vi "GT Set Capture Mode.vi"(8 "error in (no error)":errorcluster caption="错误输入（无错误）", 9 "mode":i16, 10 "encoder":i16, 11 "cardNum":i16) -> (0 "error out":errorcluster caption="错误输出", 3 "function return":i16)   [LabVIEW 2014, in "gts.lvlib"]
doc: "GT_API GT_SetCaptureMode(short cardNum,short encoder,short mode);"
uses:
  gts.lvlib
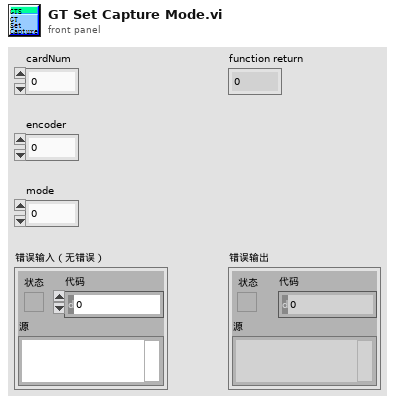
[diagram p1: front panel]
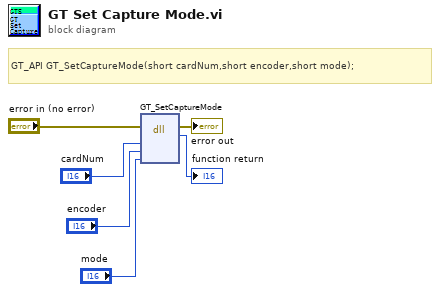
[diagram p0: block diagram]
diagram:
  # "GT_API GT_SetCaptureMode(short cardNum,short encoder,short mode);"
  n1 = dll-call lib="PTH2habs D固高科技资料GTS控制卡GTS卡18年上半年资料dllVC32bit\nmulti_cardgts.*" fn="GT_SetCaptureMode"(error in="error in (no error)", "cardNum"="cardNum", "encoder"="encoder", "mode"="mode") -> (error out=→"error out":errorcluster, →"function return":i16)  [unwired: 5 in, 1 out]
